vi "Dir Motors.vi"(1 "Direction 2":T2) -> (0 "A":T1)   [LabVIEW 2015]
uses:
  DIR GAME.ctl
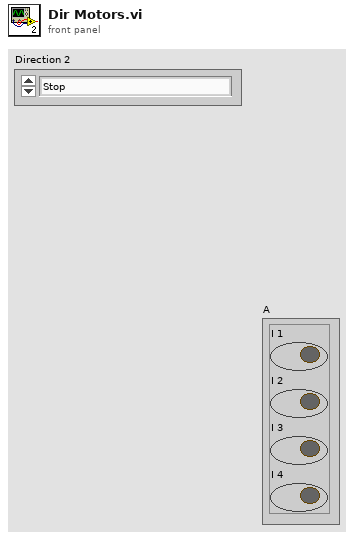
[diagram p1: front panel]
types:
  T1 = cluster{"I 1":bool, "I 2":bool, "I 3":bool, "I 4":bool}
  T2 = typedef "DIR GAME.ctl" = enum16{"Stop", "Front", "FR", "Right", "BR", "Back", "BL", "Left", "FL"}
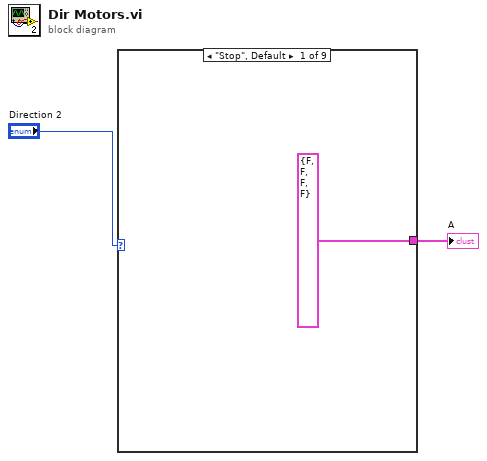
[diagram p0: block diagram]
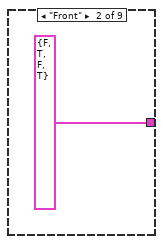
[diagram p2: hidden frame]
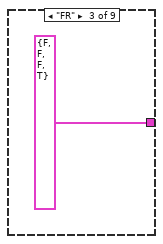
[diagram p3: hidden frame]
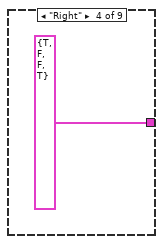
[diagram p4: hidden frame]
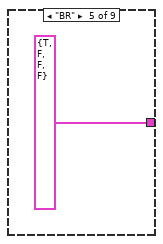
[diagram p5: hidden frame]
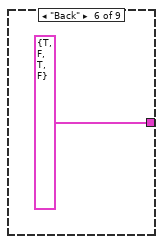
[diagram p6: hidden frame]
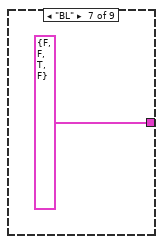
[diagram p7: hidden frame]
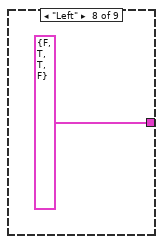
[diagram p8: hidden frame]
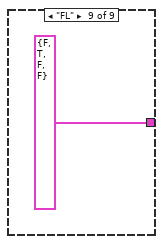
[diagram p9: hidden frame]
diagram:
  n1 = case shown="\"Stop\", Default" "Direction 2" {
    tunnel: [T1 {"I 1"=FALSE, "I 2"=FALSE, "I 3"=FALSE, "I 4"=FALSE} ("A 2") T1 {"I 1"=FALSE, "I 2"=TRUE, "I 3"=FALSE, "I 4"=TRUE} ("A 2") T1 {"I 1"=FALSE, "I 2"=FALSE, "I 3"=FALSE, "I 4"=TRUE} ("A 2") T1 {"I 1"=TRUE, "I 2"=FALSE, "I 3"=FALSE, "I 4"=TRUE} ("A 2") T1 {"I 1"=TRUE, "I 2"=FALSE, "I 3"=FALSE, "I 4"=FALSE} ("A 2") T1 {"I 1"=TRUE, "I 2"=FALSE, "I 3"=TRUE, "I 4"=FALSE} ("A 2") T1 {"I 1"=FALSE, "I 2"=FALSE, "I 3"=TRUE, "I 4"=FALSE} ("A 2") T1 {"I 1"=FALSE, "I 2"=TRUE, "I 3"=TRUE, "I 4"=FALSE} ("A 2") T1 {"I 1"=FALSE, "I 2"=TRUE, "I 3"=FALSE, "I 4"=FALSE} ("A 2")] -> w1
    frame "Stop", Default {
    }
    frame "Front" {
    }
    frame "FR" {
    }
    frame "Right" {
    }
    frame "BR" {
    }
    frame "Back" {
    }
    frame "BL" {
    }
    frame "Left" {
    }
    frame "FL" {
    }
  }
  "A" <- w1
